vi "VD-getWholeDataSet.vi"(8 "error in (no error)":errorcluster, 11 "VD-LV-LiteVNA in":refnum<class "VD-LV-LiteVNA.lvclass">) -> (0 "error out":errorcluster, 1 "Valid Data?":bool, 2 "VNA data":T1, 3 "VD-LV-LiteVNA out":refnum<class "VD-LV-LiteVNA.lvclass">, 4 "data status":T2)   [LabVIEW 2020, in "VD-LV-LiteVNA.lvclass"]
uses:
  VD-LV-LiteVNA.lvclass
  VD-data_read_status.ctl
  VD-VNA_data.ctl
  VD-action.ctl
  VD-LV-LiteVNA.lvclass/VD-LV-LiteVNA.ctl
  hardware-protocol/serial/HP-S-Serial.lvclass
panel:
  out "ms":u32
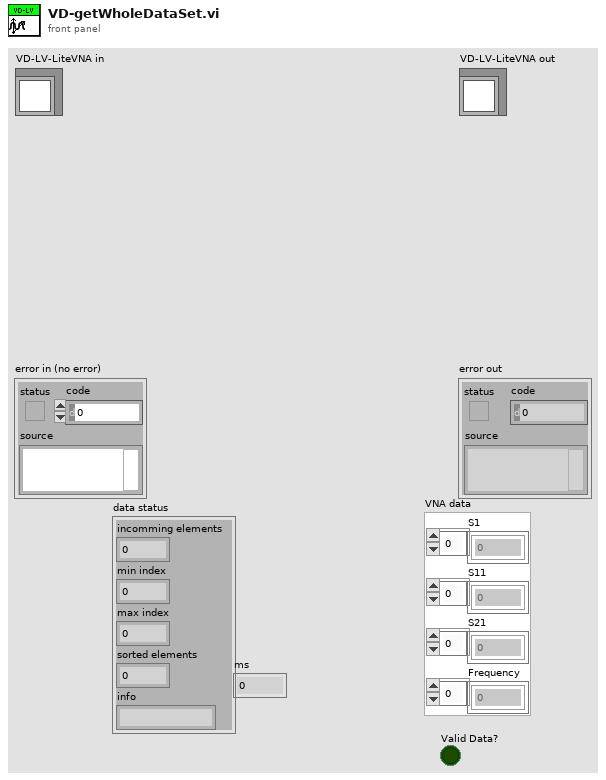
[diagram p1: front panel]
types:
  T1 = typedef "VD-LV-LiteVNA.lvclass/VD-VNA_data.ctl" = cluster{"S1":cdb[], "S11":cdb[], "S21":cdb[], "Frequency":u64[]}
  T2 = typedef "VD-LV-LiteVNA.lvclass/VD-data_read_status.ctl" = cluster{"incomming elements":i32, "min index":u16, "max index":u16, "sorted elements":i32, "info":string}
  T3 = typedef "VD-LV-LiteVNA.lvclass/VD-action.ctl" = enum16{"checkCom", "SweepStartHz", "SweepStopHz", "SweepPoints", "valuesPerFrequency", "RawSamplesMode", "ValuesFIFO", "deviceVariant", "protocolVersion", "hardwareRevision", "firmwareMajor", "firmwareMinor"}
  T4 = typedef "HP-S-Serial.lvclass/HP-S-data.ctl" = u8[]
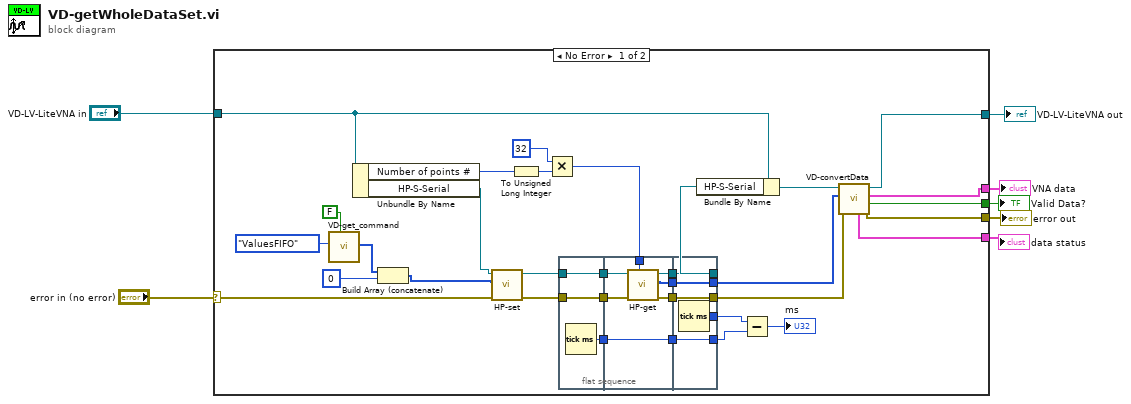
[diagram p0: block diagram]
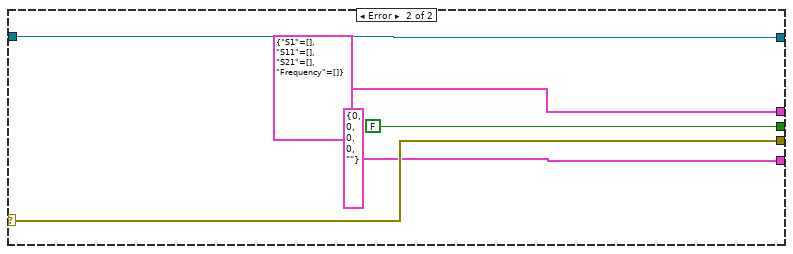
[diagram p2: hidden frame]
diagram:
  n1 = case shown="No Error" "error in (no error)" {
    selector: "error in (no error)" -> [w13 w60]
    tunnel: [w40 w60] -> w6
    tunnel: [w39 w59] -> w4
    tunnel: "VD-LV-LiteVNA in" -> [w8 w59]
    tunnel: [w38 FALSE ("Valid Data?")] -> w3
    tunnel: [w37 T2 {"incomming elements"=0, "min index"=0, "max index"=0, "sorted elements"=0, "info"=""} ("data status")] -> w2
    tunnel: [w36 T1 {"S1"=[], "S11"=[], "S21"=[], "Frequency"=[]} ("VNA data")] -> w1
    frame No Error {
      n2 = call "VD-get_command.vi"("Write?"=FALSE, "action"=VD-action."ValuesFIFO") -> ("Command"=w28:T4)  [unwired: 9 in]
      n3 = Unbundle By Name(w8) -> ("Number of points #"=w9:u16, "HP-S-Serial"=w25:refnum<class "HP-S-Serial.lvclass">)
      n4 = Build Array (concatenate)(w28, u8 0 ("x")) -> (w24:T4)
      n5 = call-dynamic "HP-set.vi"("error in (no error)"=w13, "write buffer"=w24, "HP-S-Serial in"=w25) -> ("error out"=w23:errorcluster, "HP-S-Serial out"=w22:refnum<class "HP-S-Serial.lvclass">)  [unwired: 7 in]
      n6 = To Unsigned Long Integer(number=w9) -> (unsigned 32bit integer=w18:u32)
      n7 = Multiply(x=u32 32, y=w18) -> (x*y=w19:u32)
      n8 = flat-sequence {
        tunnel: w22 -> [w42]
        tunnel: w23 -> [w43]
        tunnel: [w43] -> w35
        tunnel: [w42] -> w34
        tunnel: [w41] -> w33
        tunnel: w19 -> [w45]
        tunnel: [w48] -> w32
        tunnel: [w47] -> w31
        tunnel: [w46] -> w30
        tunnel: w35 -> [w50]
        tunnel: w34 -> [w49]
        tunnel: [w44] -> w29
        tunnel: w33 -> [w44]
        tunnel: [w53] -> w10
        tunnel: [w54] -> w11
        tunnel: [w55] -> w21
        tunnel: w32 -> [w55]
        tunnel: w31 -> [w54]
        tunnel: w30 -> [w53]
        tunnel: w29 -> [w51]
        tunnel: [w52] -> w16
        tunnel: [w51] -> w17
        frame #0 {
          n9 = Tick Count (ms)() -> (millisecond timer value=w41:u32)
        }
        frame #1 {
          n10 = call-dynamic "HP-get.vi"("get byte count"=w45, "error in (no error)"=w50, "HP-S-Serial in"=w49) -> ("error out"=w46:errorcluster, "read buffer"=w47:T4, "HP-S-Serial out"=w48:refnum<class "HP-S-Serial.lvclass">)  [unwired: 6 in]
        }
        frame #2 {
          n11 = Tick Count (ms)() -> (millisecond timer value=w52:u32)
        }
      }
      n12 = Bundle By Name(cluster=w8, "HP-S-Serial"=w21) -> (w12:refnum<class "VD-LV-LiteVNA.lvclass">)
      n13 = Subtract(x=w16, y=w17) -> (x-y=→"ms":u32)
      n14 = call-dynamic "VD-convertData.vi"("error in (no error)"=w10, "read buffer"=w11, "VD-LV-LiteVNA in"=w12) -> ("error out"=w40:errorcluster, "Valid Data?"=w38:bool, "VNA data"=w36:T1, "VD-LV-LiteVNA out"=w39:refnum<class "VD-LV-LiteVNA.lvclass">, "data status"=w37:T2)  [unwired: 4 in]
    }
    frame Error {
    }
  }
  "error out" <- w6
  "VD-LV-LiteVNA out" <- w4
  "Valid Data?" <- w3
  "data status" <- w2
  "VNA data" <- w1
